vi "Navigation_Main_position_testing april 18th.vi"() -> ()   [LabVIEW 2015]
uses:
  <vilib>/myRIO/Instrument Drivers/Onboard IO/PWM/typedefs/PWM Reference.ctl
  <vilib>/myRIO/Common/Instrument Driver Framework/Utilities/typedefs/myRIO Generic Hardware Reference.ctl
  <vilib>/myRIO/Common/Instrument Driver Framework/Utilities/typedefs/Hardware Version Enum.ctl
  <vilib>/myRIO/Common/Instrument Driver Framework/Utilities/typedefs/myRIO v1.0 Reference.ctl
  <vilib>/myRIO/Common/Instrument Driver Framework/Utilities/typedefs/Generic FPGA Reference.ctl
  <vilib>/myRIO/Common/Instrument Driver Framework/myRIO v1.0/PWM/typedefs/PWM Channels Enum.ctl
  <vilib>/myRIO/Instrument Drivers/Onboard IO/PWM/typedefs/PWM Configuration.ctl
  <vilib>/userdefined/High Color/nirio_resource_hc.ctl
  <vilib>/myRIO/Common/Instrument Driver Framework/myRIO v1.0/PWM/vis/myRIO v1.1 Open PWM.vi
  <vilib>/myRIO/Common/Instrument Driver Framework/Utilities/vis/Validate Channels.vi
  <vilib>/myRIO/Common/Instrument Driver Framework/myRIO v1.0/PWM/vis/myRIO v1.0 Reserve PWM.vi
  <vilib>/myRIO/Common/Instrument Driver Framework/myRIO v1.0/PWM/vis/myRIO v1.0 Build MUX Configuration PWM.vi
  <vilib>/myRIO/Common/Instrument Driver Framework/myRIO v1.0/Resource Manager/vis/myRIO v1.0 Reserve Channel List.vi
  <vilib>/myRIO/Common/Instrument Driver Framework/myRIO v1.0/Resource Manager/vis/myRIO v1.0 Create Configuration List.vi
  <vilib>/myRIO/Common/Instrument Driver Framework/myRIO v1.0/Resource Manager/vis/myRIO v1.0 Reserve Channel.vi
  <vilib>/myRIO/Common/Instrument Driver Framework/myRIO v1.0/Resource Manager/vis/myRIO v1.0 Unreserve Channel.vi
  <vilib>/myRIO/Common/Instrument Driver Framework/myRIO v1.0/Resource Manager/vis/myRIO v1.0 Build Mutex Name.vi
  <vilib>/FPGAPlugInAG/myRIO-1900/niLvFpga_Open_myRIO-1900.vi
  <vilib>/rvi/interface/common/dynamic/niFpgaDynamicAddResources.vi
  <vilib>/myRIO/Common/Instrument Driver Framework/Utilities/vis/FPGA Ref Manager.vi
  <vilib>/Utility/error.llb/Error Cluster From Error Code.vi
  <vilib>/myRIO/Common/Instrument Driver Framework/Utilities/vis/Ref Counter.vi
  <vilib>/rvi/errors/niLvFpgaAdjustHostInterfaceError.vi
  <vilib>/Utility/VariantDataType/GetNumericInfo.vi
  <vilib>/myRIO/Common/Instrument Driver Framework/myRIO v1.0/myRIO v1.1 Open.vi
  <vilib>/myRIO/Common/Instrument Driver Framework/Utilities/vis/IO Manager.vi
  <vilib>/myRIO/Common/Instrument Driver Framework/Utilities/vis/Configuration Manager.vi
  <vilib>/myRIO/Common/Instrument Driver Framework/myRIO v1.0/Resource Manager/vis/myRIO v1.0 Configure IO.vi
  <vilib>/myRIO/Common/Instrument Driver Framework/myRIO v1.0/myRIO v1.0 Close.vi
  <vilib>/myRIO/Common/Instrument Driver Framework/myRIO v1.0/PWM/vis/myRIO v1.0 Write PWM.vi
  <vilib>/addons/control/pid/pid.llb/PID (DBL).vi
  <vilib>/rvi/interface/nirviOpenFPGA/nirviOpenFPGA.xnode
  Navi/E/FPGA Bitfiles/NavigationProjec_FPGATarget2_FPGAMainNavigati_PWPHW8gwDxI.lvbitx
  <vilib>/rvi/interface/nirviReadWriteControl/nirviReadWriteControl.xnode
  <vilib>/myRIO/Instrument Drivers/Onboard IO/PWM/vis/myRIO PWM Open.xnode
  <vilib>/myRIO/Instrument Drivers/Onboard IO/PWM/PWM.lvlib
  <vilib>/myRIO/Instrument Drivers/Utilities/Utilities.lvlib
  NiFpgaLv.dll
  <vilib>/rvi/interface/Simulation/niFpgaSimulationCallBeginRW.vi
  <vilib>/addons/control/pid/NI_PID_pid.lvlib
panel:
  out "right 2":dbl
  out "left 2":dbl
  in  "right ctrl":dbl min=-0.133 max=0.133 step=0.01
  in  "left ctrl":dbl min=-0.133 max=0.133 step=0.01
  in  "reset start position":bool=TRUE
  in  "theta goal":dbl=10.0
  in  "y goal":dbl=10.0
  out "stop switch":dbl=1.0
  out "distance to goal":dbl
  out "loc_y":dbl
  out "loc_x":dbl
  out "loc_theta":dbl
  out "start y":dbl
  out "start angle":dbl=1.0
  out "start x":dbl=1.0
  in  "set start position":bool=TRUE
  out "goal reached":bool=TRUE
  out "x/y":dbl
  out "scale":dbl=1.0
  in  "x goal":dbl=10.0
  in  "L Desired Input Velocity (ft/s) 4":dbl(knob) scale=-4.0..4.0
  in  "R Min Linear Velocity (ft/s)  2":dbl=-2.0 format="%#_13g"
  in  "L Min Linear Velocity (ft/s) 9":dbl=-2.0 format="%#_13g"
  in  "R Max Linear Velocity (ft/s) 5":dbl=2.0 format="%#_13g"
  in  "L Max Linear Velocity (ft/s) 5":dbl=2.0 format="%#_13g"
  in  "R Desired Input Velocity (ft/s) 5":dbl(knob) scale=-4.0..4.0
  out "left":dbl
  out "right":dbl
  out "left wheels actual pwm":dbl
  in  "stop 3":bool
  out "left pwm":dbl(graph)
  out "dt out (s) 3":dbl format="%.3f"
  in  "output range 3":cluster{"output high":dbl, "output low":dbl}={"output high"=0.13333, "output low"=-0.13333} {"output low" format="%.6f"; "output high" format="%.5f"}
  in  "PID gains 3":T1={"proportional gain (Kc)"=0.002, "integral time (Ti, min)"=7e-07, "derivative time (Td, min)"=0.0} {"derivative time (Td, min)" format="%.8f"; "integral time (Ti, min)" format="%.8f"; "proportional gain (Kc)" format="%.8f"}
  out "desired pwm 2":dbl
  out "feedback 2":dbl
  out ".not. x? 3":bool
  out "Elapsed Time (s) 2":dbl caption="Elapsed Time (s)"
  out "x traveled 2":dbl
  out "y traveled 2":dbl
  out "avg 124":dbl
  out "avg 457":dbl
  out "psi dot 2":dbl
  out "distance traveled 2":dbl
  out "y dot 2":dbl
  out "x dot 2":dbl
  out "x position 2":dbl
  out "y position 2":dbl
  out "reset x y 2":dbl
  out "Tick Count(mSec) 2":u32 caption="Tick Count(mSec)"
  in  "start y 2":dbl=3.0
  in  "start x 2":dbl=1.0
  out "right wheels actual pwm":dbl
  in  "stop 2":bool
  out "right pwm":dbl(graph)
  out "dt out (s) 2":dbl format="%.3f"
  in  "output range 2":cluster{"output high":dbl, "output low":dbl}={"output high"=0.13333, "output low"=-0.13333} {"output low" format="%.6f"; "output high" format="%.5f"}
  in  "PID gains 2":T1={"proportional gain (Kc)"=0.002, "integral time (Ti, min)"=7e-07, "derivative time (Td, min)"=0.0} {"derivative time (Td, min)" format="%.8f"; "integral time (Ti, min)" format="%.8f"; "proportional gain (Kc)" format="%.8f"}
  out "desired pwm":dbl
  out "feedback":dbl
  out ".not. x? 2":bool
  out "Elapsed Time (s)":dbl
  out "LF Rot Velocity (rot/s)":dbl
  out "LM Rot Velocity (rot/s)":dbl
  out "LR Rot Velocity (rot/s)":dbl
  out "RR Rot Velocity (rot/s)":dbl
  out "RM Linear Velocity (rot/s)":dbl
  out "RF Linear Velocity (rot/s)":dbl
  in  "Encoder Reset":bool
  out "SYS.SELECTA":u8 format="%08b"
  out "ENC.B_c.CNTR":i32
  out "ENC.B_b.CNTR":i32
  out "ENC.B_a.CNTR":i32
  out "ENC.A_c.CNTR":i32
  out "ENC.A_b.CNTR":i32
  out "ENC.A_a.CNTR":i32
  in  "R Min Linear Velocity (ft/s)":dbl=-2.0 format="%#_13g"
  in  "R Max Linear Velocity (ft/s)":dbl=2.0 format="%#_13g"
  in  "L Min Linear Velocity (ft/s)":dbl=-2.0 format="%#_13g"
  in  "L Max Linear Velocity (ft/s)":dbl=2.0 format="%#_13g"
  out "Current Rot Velocity (rot/s)":T2(graph)
  # "starts the loop"
  # "Motor Control Parameters"
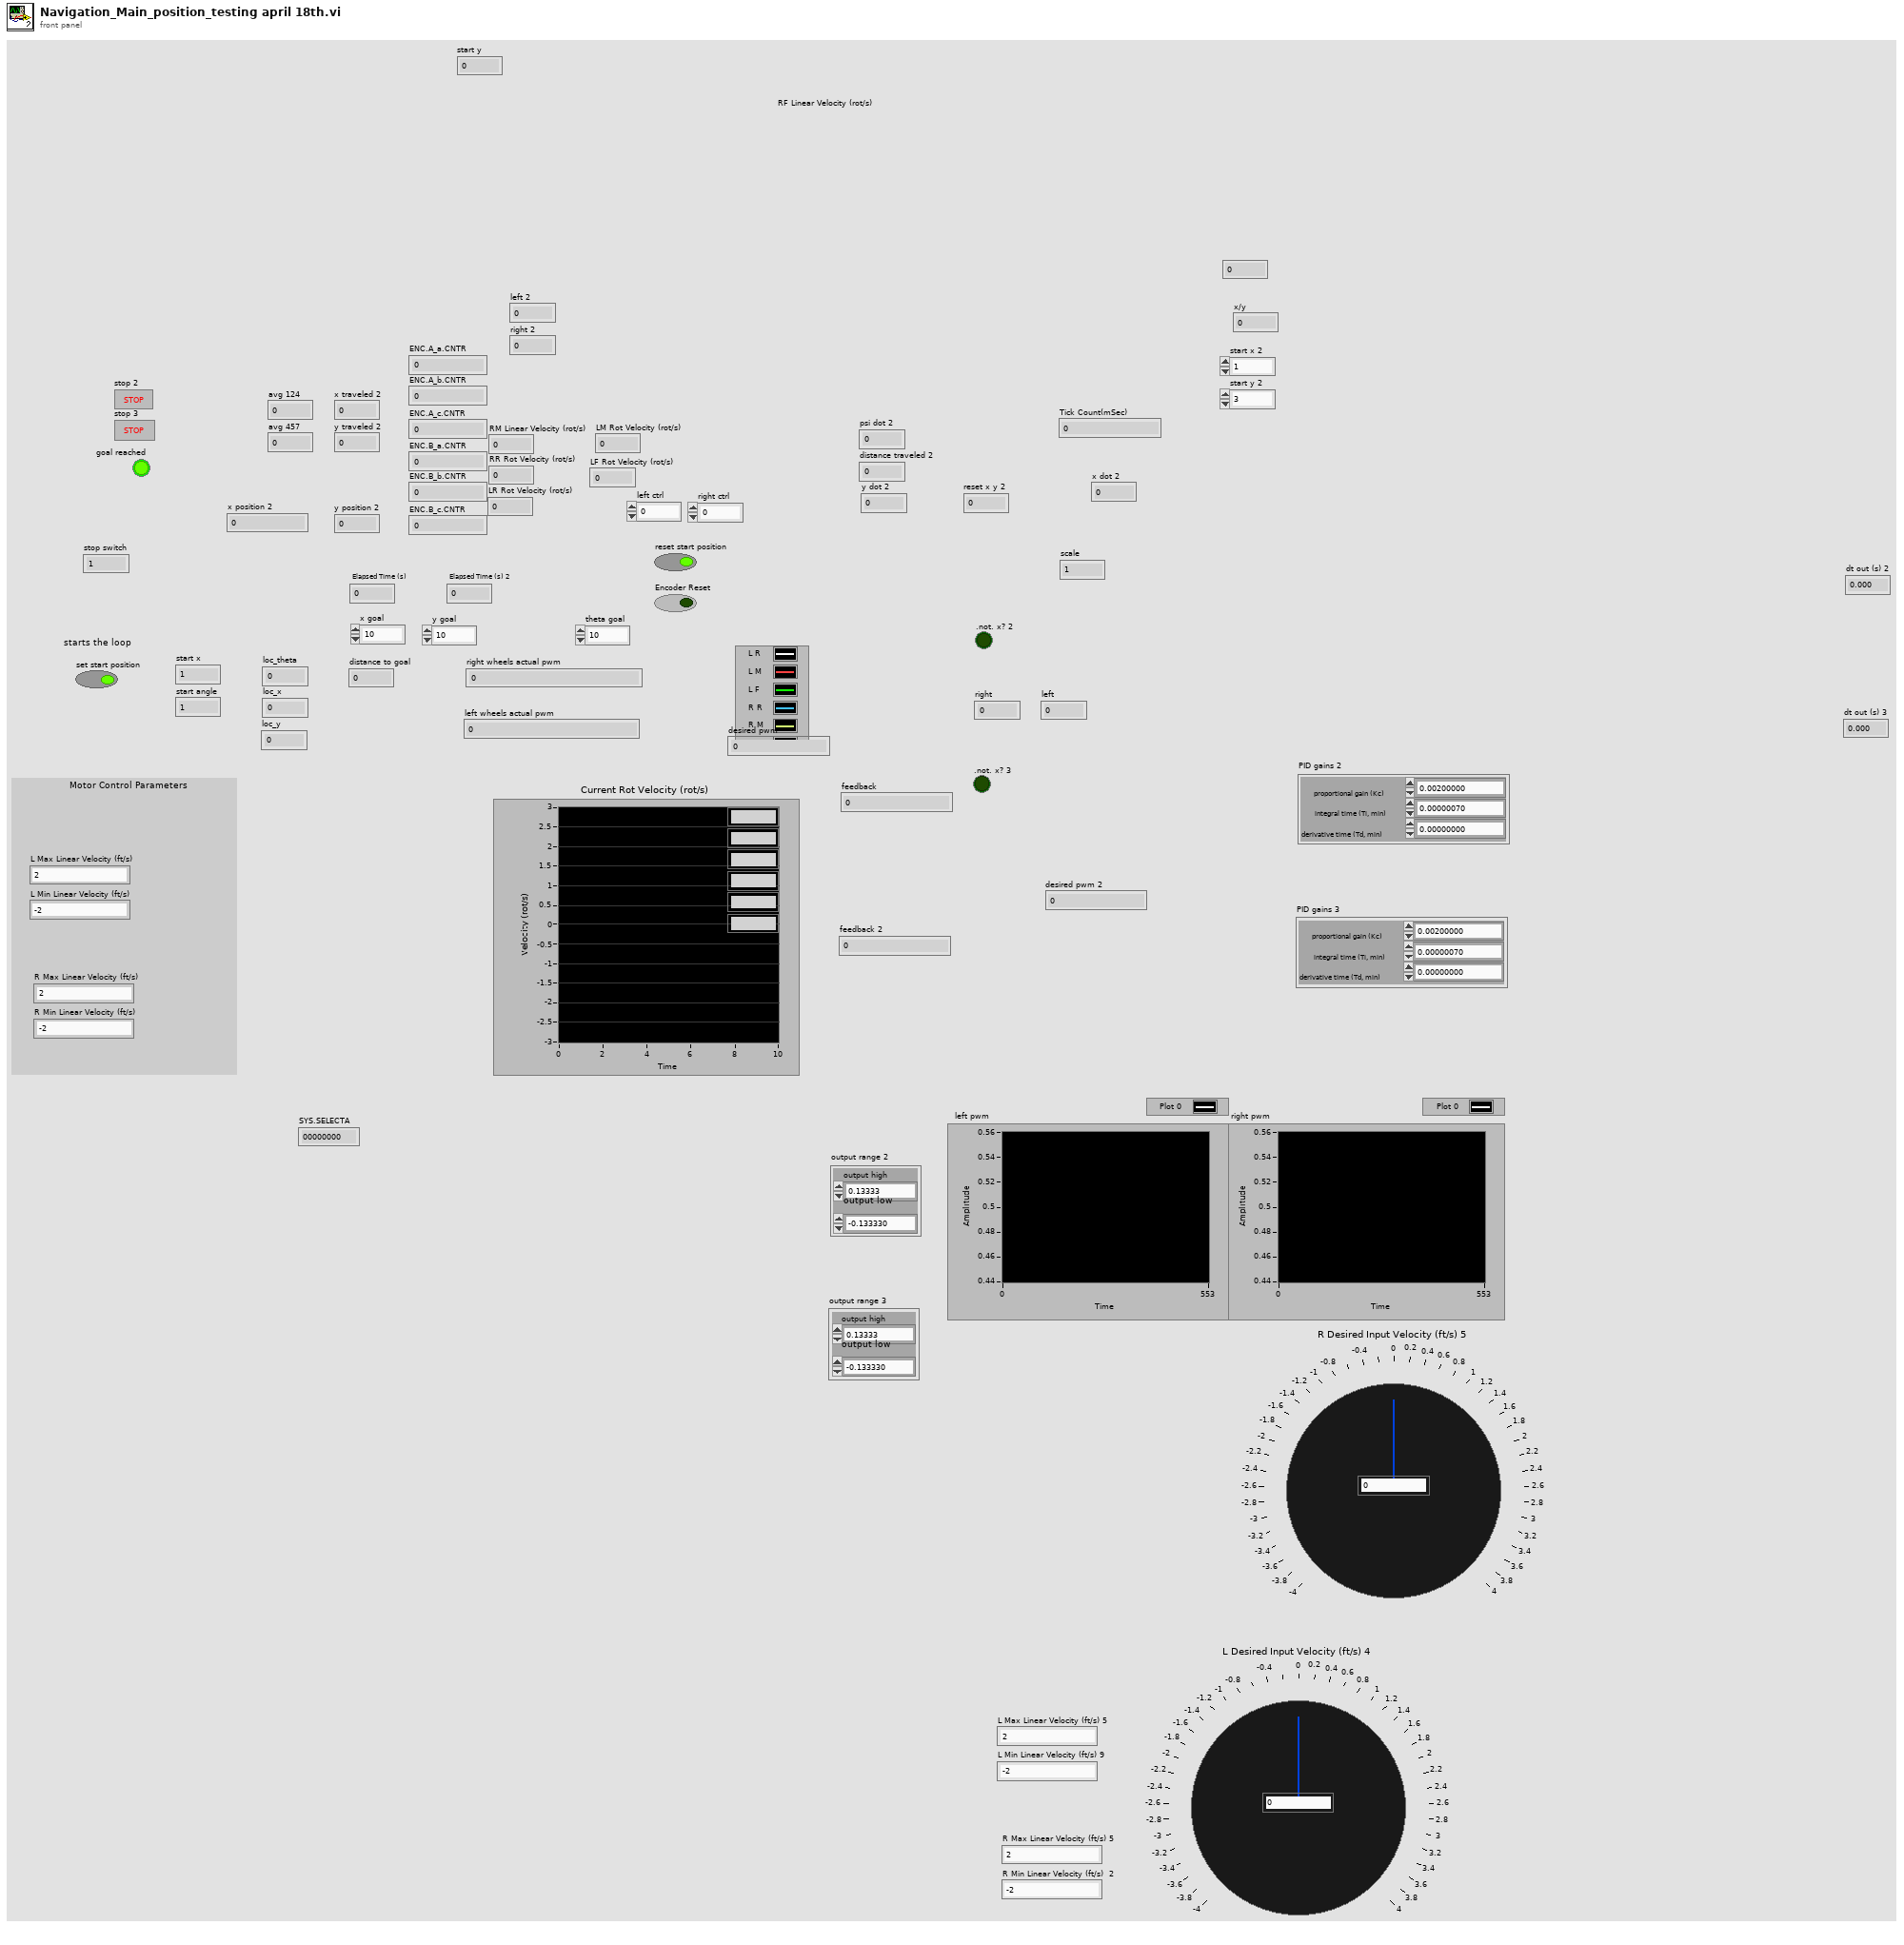
[diagram p1: front panel]
types:
  T1 = cluster{"proportional gain (Kc)":dbl, "integral time (Ti, min)":dbl, "derivative time (Td, min)":dbl}
  T2 = cluster{"Rotational Velocity (RPS)":dbl, "Rotational Velocity (RPS)":dbl, "Rotational Velocity (RPS)":dbl, "Rotational Velocity (RPS)":dbl, "Rotational Velocity (RPS)":dbl, "Rotational Velocity (RPS)":dbl}
  T3 = typedef "nirio_resource_hc.ctl" = tag
  T4 = typedef "Hardware Version Enum.ctl" = enum16{"Unknown", "myRIO-1900", "myRIO-1950", "roboRIO"}
  T5 = typedef "PWM.lvlib/PWM Reference.ctl" = cluster{"myRIO Reference":T6, "PWM Channels Enum":T9, "PWM Configuration":T10}
  T6 = typedef "myRIO Generic Hardware Reference.ctl" = cluster{"myRIO Model":T4, "myRIO Hardware Reference":T7}
  T7 = typedef "myRIO v1.0 Reference.ctl" = cluster{"Generic FPGA Reference":T8, "Allow multiple opens":bool}
  T8 = typedef "Generic FPGA Reference.ctl" = refnum<k20>
  T9 = typedef "PWM Channels Enum.ctl" = enum16{"Not Connected", "C/PWM0", "C/PWM1", "A/PWM0", "A/PWM1", "A/PWM2", "B/PWM0", "B/PWM1", "B/PWM2", "PWM/PWM0", "PWM/PWM1", "PWM/PWM2", "PWM/PWM3", "PWM/PWM4", "PWM/PWM5", "PWM/PWM6", "PWM/PWM7", "PWM/PWM8", "PWM/PWM9"}
  T10 = typedef "PWM.lvlib/PWM Configuration.ctl" = cluster{"Frequency":dbl, "Duty Cycle":dbl}
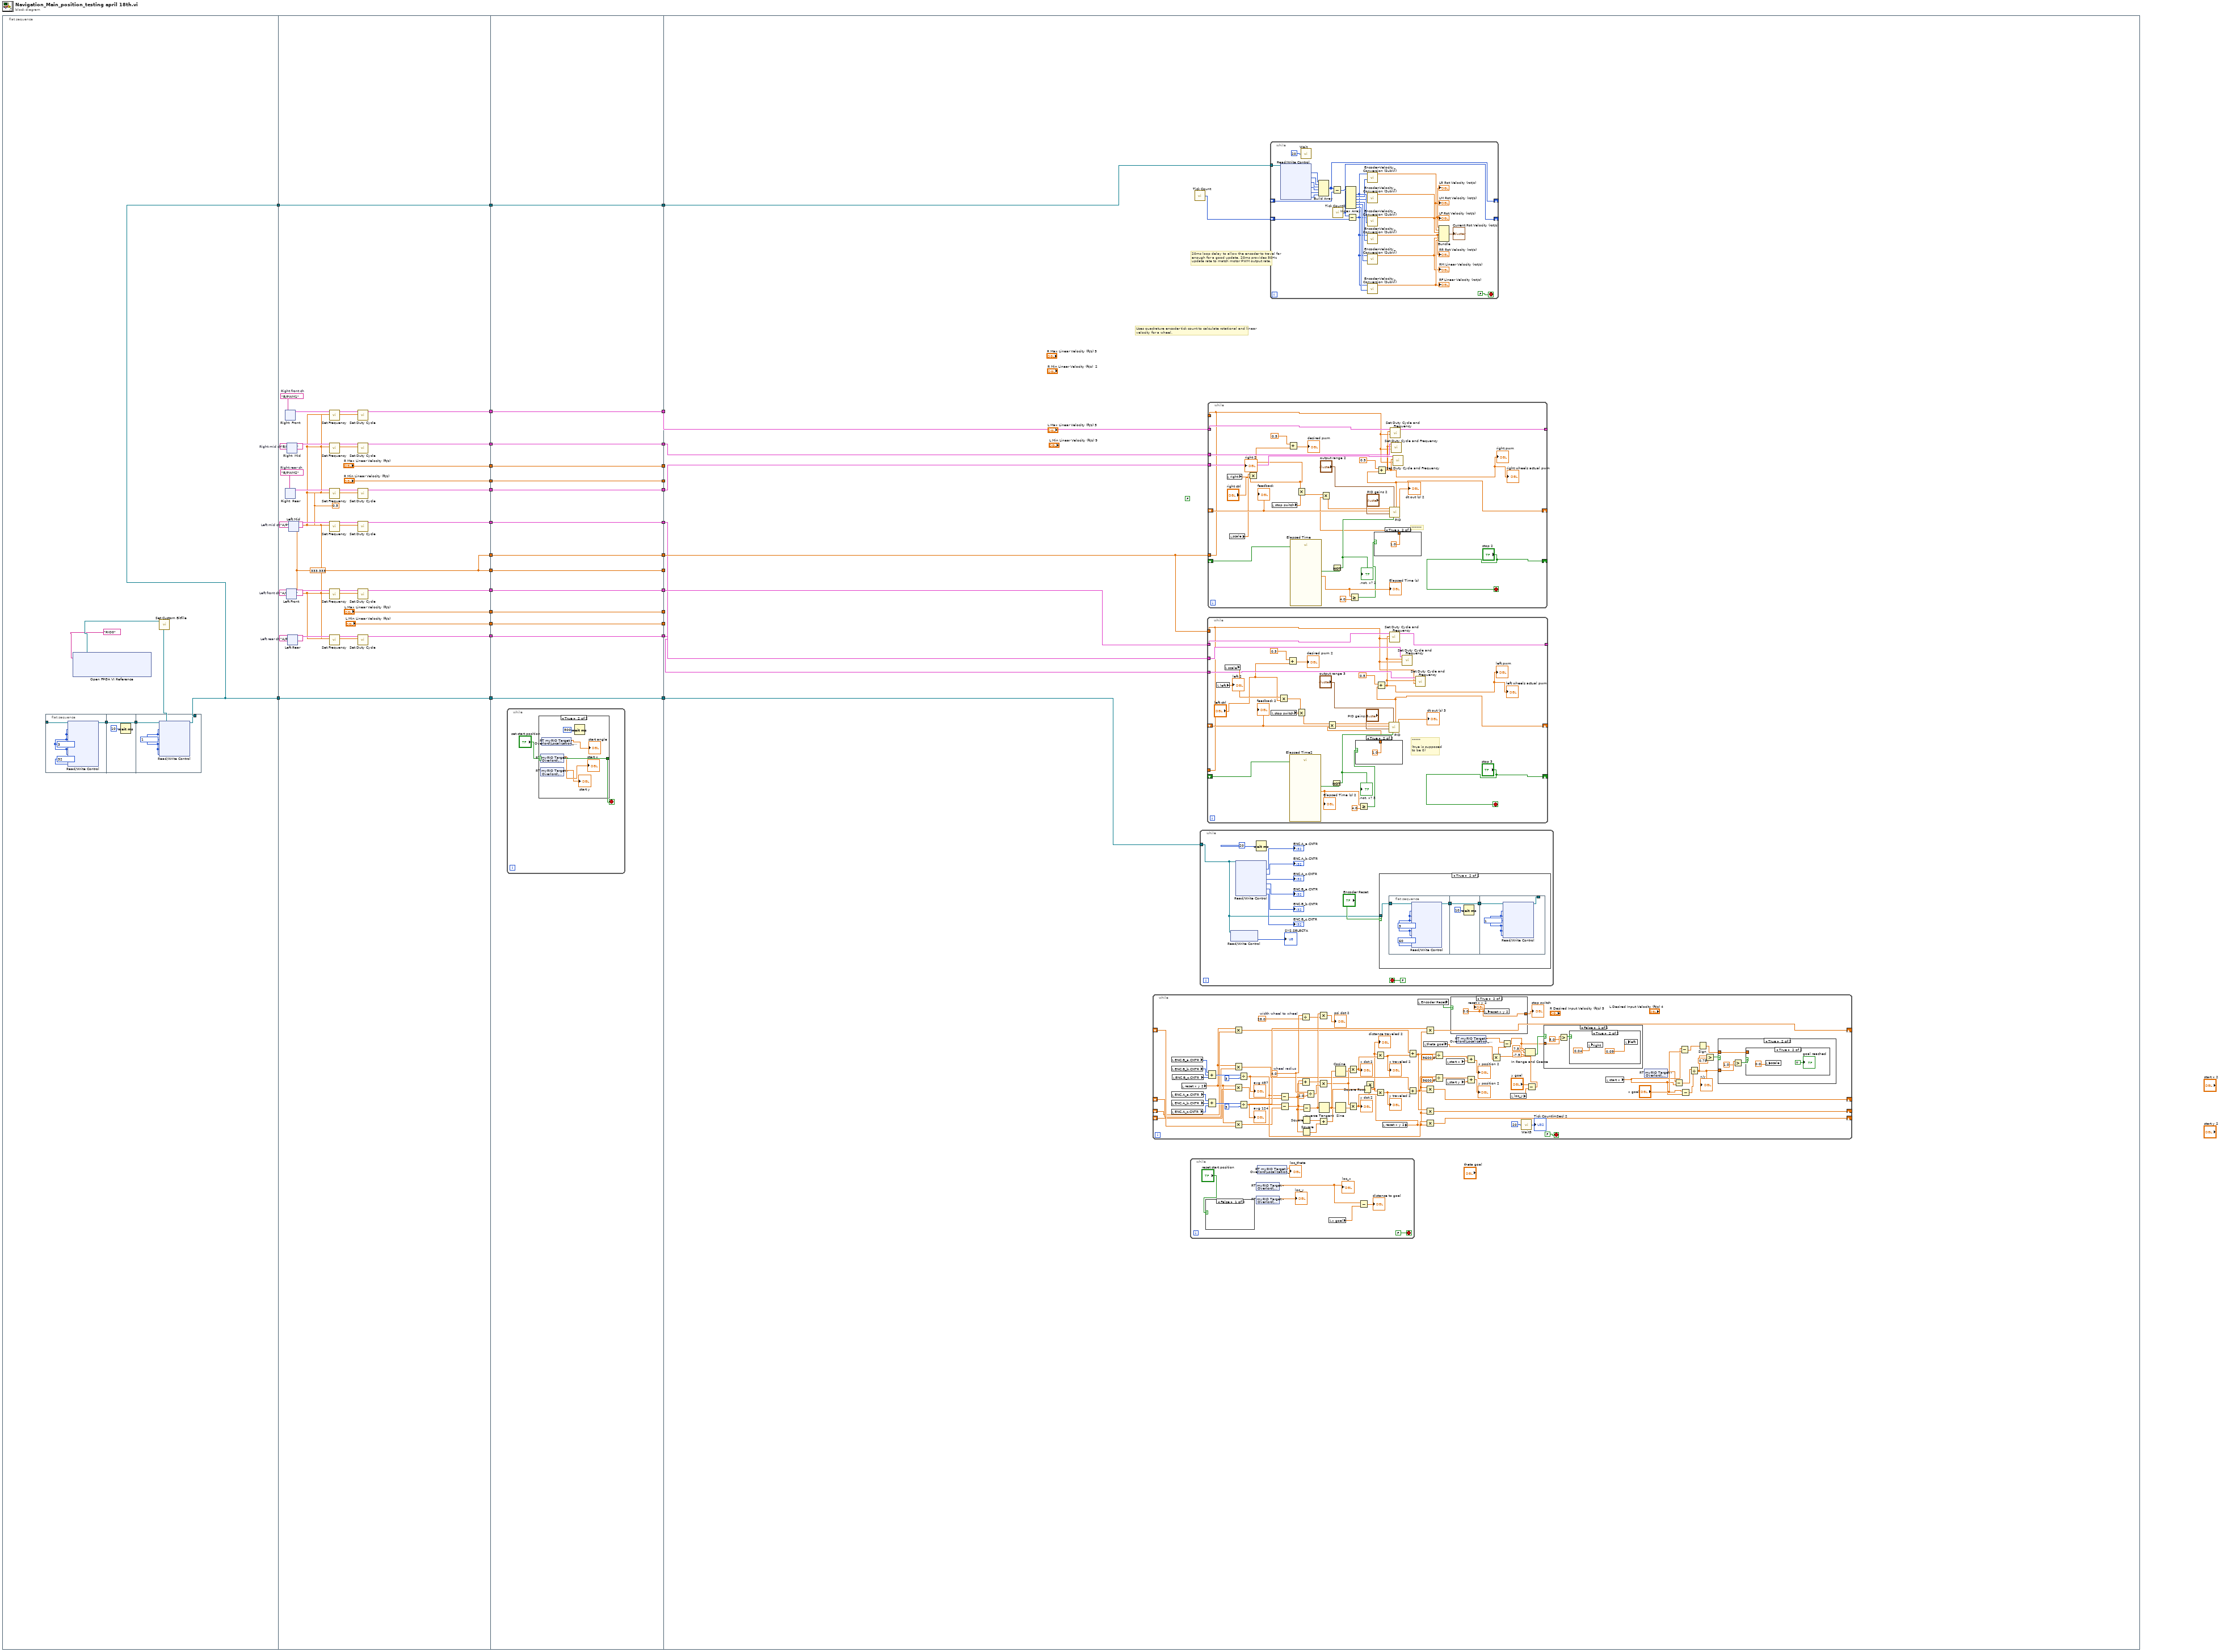
[diagram p0: block diagram]
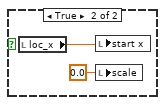
[diagram p3: hidden frame]
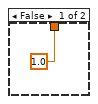
[diagram p4: hidden frame]
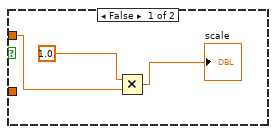
[diagram p5: hidden frame]
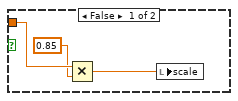
[diagram p6: hidden frame]
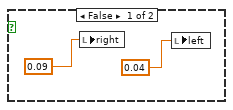
[diagram p7: hidden frame]
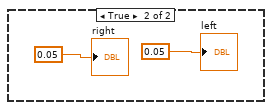
[diagram p8: hidden frame]
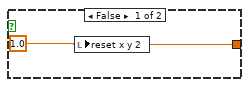
[diagram p9: hidden frame]
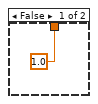
[diagram p10: hidden frame]
diagram:
  n1 = flat-sequence {
    tunnel: [w33] -> w30
    tunnel: [w33] -> w29
    tunnel: [w46] -> w28
    tunnel: [w61] -> w26
    tunnel: [w57] -> w24
    tunnel: [w56] -> w22
    tunnel: [w55] -> w20
    tunnel: [w54] -> w18
    tunnel: [w53] -> w16
    tunnel: ["L Max Linear Velocity (ft/s)"] -> w14
    tunnel: ["L Min Linear Velocity (ft/s)"] -> w12
    tunnel: ["R Max Linear Velocity (ft/s)"] -> w10
    tunnel: ["R Min Linear Velocity (ft/s)"] -> w8
    tunnel: [w48] -> w6
    tunnel: w30 -> [w47]
    tunnel: [w47] -> w4
    tunnel: w29 -> [w48]
    tunnel: [w46] -> w2
    tunnel: w28 -> [w187]
    tunnel: [w187] -> w27
    tunnel: w26 -> [w186]
    tunnel: [w186] -> w25
    tunnel: w24 -> [w185]
    tunnel: [w185] -> w23
    tunnel: w22 -> [w184]
    tunnel: [w184] -> w21
    tunnel: w20 -> [w183]
    tunnel: [w183] -> w19
    tunnel: w18 -> [w182]
    tunnel: [w182] -> w17
    tunnel: w16 -> [w181]
    tunnel: [w181] -> w15
    tunnel: w14 -> [w180]
    tunnel: [w180] -> w13
    tunnel: w12 -> [w179]
    tunnel: [w179] -> w11
    tunnel: w10 -> [w178]
    tunnel: [w178] -> w9
    tunnel: w8 -> [w177]
    tunnel: [w177] -> w7
    tunnel: w6 -> [w176]
    tunnel: [w176] -> w5
    tunnel: w4 -> [w175]
    tunnel: [w175] -> w3
    tunnel: w2 -> [w174]
    tunnel: [w174] -> w1
    tunnel: w27 -> [_]
    tunnel: w25 -> [w195]
    tunnel: w23 -> [w201]
    tunnel: w21 -> [w198]
    tunnel: w19 -> [w197]
    tunnel: w17 -> [w196]
    tunnel: w15 -> [w200]
    tunnel: w13 -> [_]
    tunnel: w11 -> [_]
    tunnel: w9 -> [_]
    tunnel: w7 -> [_]
    tunnel: w5 -> [w203]
    tunnel: w3 -> [w202]
    tunnel: w1 -> [w199]
    frame #0 {
      n2 = flat-sequence {
        tunnel: w34 -> [w39]
        tunnel: [w37] -> w36
        tunnel: w36 -> [w41]
        tunnel: [w41] -> w35
        tunnel: w35 -> [w44]
        tunnel: [w43] -> w33
        frame #0 {
          w38 = u8 32 ("SYS.SELECTA")
          w40 = u8 3 ("ENC.B_c.CNFG")
          n3 = xnode "Read/Write Control"("FPGA VI Reference In"=w39, "ENC.A_a.CNFG"=w40, "ENC.A_b.CNFG"=w40, "ENC.A_c.CNFG"=w40, "ENC.B_a.CNFG"=w40, "ENC.B_b.CNFG"=w40, "ENC.B_c.CNFG"=w40, "SYS.SELECTA"=w38, "SYS.SELECTB"=w38) -> ("FPGA VI Reference Out"=w37:refnum<k20>)  [unwired: 1 in, 1 out]
        }
        frame #1 {
          n4 = Wait (ms)(milliseconds to wait=u32 10) -> ()  [unwired: 1 out]
        }
        frame #2 {
          w45 = u8 1 ("ENC.B_c.CNFG")
          n5 = xnode "Read/Write Control"("FPGA VI Reference In"=w44, "ENC.A_a.CNFG"=w45, "ENC.A_b.CNFG"=w45, "ENC.A_c.CNFG"=w45, "ENC.B_a.CNFG"=w45, "ENC.B_b.CNFG"=w45, "ENC.B_c.CNFG"=w45) -> ("FPGA VI Reference Out"=w43:refnum<k20>)  [unwired: 1 in, 1 out]
        }
      }
      n6 = xnode "Open FPGA VI Reference"("resource name"=tag "RIO0") -> ("FPGA VI Reference Out"=w32:refnum<k20>)  [unwired: 1 in, 1 out]
      n7 = call <vilib>:"Set Custom Bitfile.vi"("Custom FPGA Reference In"=w32) -> ("Custom FPGA Reference Out"=w34:refnum<k20>)  [unwired: 9 in, 1 out]
    }
    frame #1 {
      w58 = 0.5 ("Duty Cycle")
      w46 = 333.333 ("Frequency [Hz]")
      w72 = tag "B/PWM2"  # Right rear ch
      w73 = tag "B/PWM0"  # Right mid ch
      w74 = tag "B/PWM1"  # Right front ch
      w75 = tag "A/PWM2"  # Left rear ch
      w76 = tag "A/PWM1"  # Left mid ch
      w77 = tag "A/PWM0"  # Left front ch
      n8 = xnode "Right  Front"("Channel Name"=w74) -> ("PWM Ref Out"=w68:T5)  [unwired: 2 in, 1 out]
      n9 = xnode "Right  Rear"("Channel Name"=w72) -> ("PWM Ref Out"=w66:T5)  [unwired: 2 in, 1 out]
      n10 = xnode "Left Front"("Channel Name"=w77) -> ("PWM Ref Out"=w71:T5)  [unwired: 2 in, 1 out]
      n11 = xnode "Right  Mid"("Channel Name"=w73) -> ("PWM Ref Out"=w67:T5)  [unwired: 2 in, 1 out]
      n12 = xnode "Left Rear"("Channel Name"=w75) -> ("PWM Ref Out"=w69:T5)  [unwired: 2 in, 1 out]
      n13 = xnode "Left Mid"("Channel Name"=w76) -> ("PWM Ref Out"=w70:T5)  [unwired: 2 in, 1 out]
      n14 = call <vilib>:"Set Frequency.vi"("Frequency [Hz]"=w46, "PWM Ref In"=w68) -> ("PWM Ref Out"=w62:T5)  [unwired: 7 in, 1 out]
      n15 = call <vilib>:"Set Frequency.vi"("Frequency [Hz]"=w46, "PWM Ref In"=w67) -> ("PWM Ref Out"=w63:T5)  [unwired: 7 in, 1 out]
      n16 = call <vilib>:"Set Frequency.vi"("Frequency [Hz]"=w46, "PWM Ref In"=w66) -> ("PWM Ref Out"=w64:T5)  [unwired: 7 in, 1 out]
      n17 = call <vilib>:"Set Frequency.vi"("Frequency [Hz]"=w46, "PWM Ref In"=w70) -> ("PWM Ref Out"=w59:T5)  [unwired: 7 in, 1 out]
      n18 = call <vilib>:"Set Frequency.vi"("Frequency [Hz]"=w46, "PWM Ref In"=w71) -> ("PWM Ref Out"=w65:T5)  [unwired: 7 in, 1 out]
      n19 = call <vilib>:"Set Frequency.vi"("Frequency [Hz]"=w46, "PWM Ref In"=w69) -> ("PWM Ref Out"=w60:T5)  [unwired: 7 in, 1 out]
      n20 = call <vilib>:"Set Duty Cycle.vi"("Duty Cycle"=w58, "PWM Ref In"=w62) -> ("PWM Ref Out"=w57:T5)  [unwired: 7 in, 1 out]
      n21 = call <vilib>:"Set Duty Cycle.vi"("Duty Cycle"=w58, "PWM Ref In"=w63) -> ("PWM Ref Out"=w56:T5)  [unwired: 7 in, 1 out]
      n22 = call <vilib>:"Set Duty Cycle.vi"("Duty Cycle"=w58, "PWM Ref In"=w64) -> ("PWM Ref Out"=w55:T5)  [unwired: 7 in, 1 out]
      n23 = call <vilib>:"Set Duty Cycle.vi"("Duty Cycle"=w58, "PWM Ref In"=w59) -> ("PWM Ref Out"=w54:T5)  [unwired: 7 in, 1 out]
      n24 = call <vilib>:"Set Duty Cycle.vi"("Duty Cycle"=w58, "PWM Ref In"=w65) -> ("PWM Ref Out"=w53:T5)  [unwired: 7 in, 1 out]
      n25 = call <vilib>:"Set Duty Cycle.vi"("Duty Cycle"=w58, "PWM Ref In"=w60) -> ("PWM Ref Out"=w61:T5)  [unwired: 7 in, 1 out]
    }
    frame #2 {
      n26 = while {
        stop <- w188 stop-if-true
        n27 = case shown="True" "set start position" {
          selector: "set start position" -> [_ w194]
          tunnel: [_ w194] -> w188
          frame False {
          }
          frame True {
            n28 = shared-variable "RT myRIO Target - Overlord\\Localization_Variables_r0.lvlib\\loc_x"() -> (→"start x":dbl)  [unwired: 1 in, 1 out]
            n29 = shared-variable "RT myRIO Target - Overlord\\Localization_Variables_r0.lvlib\\loc_y"() -> (→"start y":dbl)  [unwired: 1 in, 1 out]
            n30 = shared-variable "RT myRIO Target - Overlord\\Localization_Variables_r0.lvlib\\loc_theta"() -> (→"start angle":dbl)  [unwired: 1 in, 1 out]
            n31 = Wait (ms)(milliseconds to wait=u32 500) -> ()  [unwired: 1 out]
          }
        }
      }
    }
    frame #3 {
      (unwired) FALSE
      # "Uses quadrature encoder tick count to calculate rotational and linear velocity for a wheel."
      # "20ms loop delay to allow the encoder to travel far enough for a good update. 20ms provides 50Hz update rate to match motor PWM output rate."
      n32 = while {
        shift-right: [w277] -> _
        shift-left: _ -> [w315]
        shift-right: [w274] -> _
        shift-left: _ -> [w314]
        shift-right: [w276] -> _
        shift-left: _ -> [w289]
        shift-right: [w275] -> _
        shift-left: _ -> [w288]
        stop <- FALSE stop-if-true
        w310 = 28.0  # width wheel to wheel
        w311 = 4.0  # wheel radius
        n33 = local read "ENC.B_a.CNTR"() -> (w320:i32)
        n34 = local read "ENC.B_b.CNTR"() -> (w319:i32)
        n35 = local read "ENC.A_a.CNTR"() -> (w323:i32)
        n36 = local read "ENC.A_b.CNTR"() -> (w322:i32)
        n37 = local read "ENC.A_c.CNTR"() -> (w321:i32)
        n38 = local read "ENC.B_c.CNTR"() -> (w318:i32)
        n39 = local read "reset x y 2"() -> (w273:dbl)
        n40 = Compound Arithmetic op=ADD(w320, w319, w318) -> (w326:i32)
        n41 = Compound Arithmetic op=ADD(w323, w322, w321) -> (w327:i32)
        n42 = Multiply(x=w273, y=w288) -> (x*y=w279:dbl)
        n43 = Multiply(x=w273, y=w289) -> (x*y=w280:dbl)
        n44 = Multiply(x=w273, y=w314) -> (x*y=w278:dbl)
        n45 = Multiply(x=w273, y=w315) -> (x*y=w281:dbl)
        n46 = Divide(x=w326, y=3) -> (x/y=w313:dbl)
        "avg 457" <- w313
        n47 = Divide(x=w327, y=3) -> (x/y=w316:dbl)
        "avg 124" <- w316
        n48 = Subtract(x=w313, y=w278) -> (x-y=w303:dbl)
        n49 = Subtract(x=w316, y=w281) -> (x-y=w304:dbl)
        n50 = Divide(x=w311, y=w310) -> (x/y=w306:dbl)
        n51 = Add(x=w304, y=w303) -> (x+y=w308:dbl)
        n52 = Square(x=w304) -> (x^2=w301:dbl)
        n53 = Square(x=w303) -> (x^2=w302:dbl)
        n54 = Subtract(x=w304, y=w303) -> (x-y=w307:dbl)
        n55 = Divide(x=w311, y=2.0) -> (x/y=w309:dbl)
        n56 = Multiply(x=w307, y=w306) -> (x*y=→"psi dot 2":dbl)
        n57 = Multiply(x=w308, y=w309) -> (x*y=w297:dbl)
        n58 = Add(x=w301, y=w302) -> (x+y=w300:dbl)
        n59 = Inverse Tangent(1:w307) -> (0:w305:dbl)
        n60 = Cosine(x=w305) -> (cos(x)=w298:dbl)
        n61 = Sine(x=w305) -> (sin(x)=w299:dbl)
        n62 = Multiply(x=w297, y=w298) -> (x*y=w295:dbl)
        "x dot 2" <- w295
        n63 = Multiply(x=w297, y=w299) -> (x*y=w296:dbl)
        "y dot 2" <- w296
        n64 = Square Root(x=w300) -> (sqrt(x)=w294:dbl)
        n65 = local read "reset x y 2"() -> (w271:dbl)
        n66 = Multiply(x=w294, y=w271) -> (x*y=w272:dbl)
        "distance traveled 2" <- w272
        n67 = Multiply(x=w272, y=w295) -> (x*y=w293:dbl)
        "x traveled 2" <- w293
        n68 = Multiply(x=w272, y=w296) -> (x*y=w292:dbl)
        "y traveled 2" <- w292
        n69 = Add(x=w279, y=w293) -> (x+y=w291:dbl)
        n70 = Add(x=w280, y=w292) -> (x+y=w283:dbl)
        n71 = local read "Encoder Reset"() -> (w270:bool)
        n72 = local read "theta goal"() -> (w251:dbl)
        n73 = Multiply(x=w316, y=w271) -> (x*y=w277:dbl)
        n74 = Multiply(x=w271, y=w283) -> (x*y=w276:dbl)
        n75 = Multiply(x=w291, y=w271) -> (x*y=w275:dbl)
        n76 = Multiply(x=w313, y=w271) -> (x*y=w274:dbl)
        n77 = Divide(x=w291, y=9600.0) -> (x/y=w286:dbl)
        n78 = Divide(x=w283, y=9600.0) -> (x/y=w287:dbl)
        n79 = local read "start x"() -> (w284:dbl)
        n80 = local read "start y"() -> (w285:dbl)
        n81 = case shown="True" w270 {
          tunnel: [w350 w351] -> w252
          frame False {
            w350 = 1.0
            n82 = local write "reset x y 2"(w350) -> ()
          }
          frame True {
            w351 = 0.0
            n83 = local write "reset x y 2"(w351) -> ()
            "reset x y 2" <- w351
          }
        }
        "stop switch" <- w252
        n84 = shared-variable "RT myRIO Target - Overlord\\Localization_Variables_r0.lvlib\\loc_theta"() -> (w250:dbl)  [unwired: 1 in, 1 out]
        n85 = Add(x=w286, y=w284) -> (x+y=→"x position 2":dbl)
        n86 = Add(x=w287, y=w285) -> (x+y=→"y position 2":dbl)
        n87 = local read "loc_y"() -> (w246:dbl)
        n88 = call "Wait3"("Count(mSec)"=u32 20) -> ("Tick Count(mSec)"=→"Tick Count(mSec) 2":u32)
        n89 = Subtract(x="y goal", y=w246) -> (x-y=w245:dbl)
        n90 = Multiply(x=w245, y=w251) -> (x*y=w248:dbl)
        n91 = Subtract(x=w250, y=w248) -> (x-y=w249:dbl)
        n92 = In Range and Coerce(upper limit=7.5, x=w249, lower limit=-7.5) -> (In Range?=w264:bool)  [unwired: 1 out]
        n93 = case shown="False" w264 {
          tunnel: w249 -> [w343 _]
          frame False {
            n94 = Greater?(x=w343, y=5.0) -> (0:w341:bool)
            n95 = case shown="True" w341 {
              frame False {
                n96 = local write "right"(0.09) -> ()
                n97 = local write "left"(0.04) -> ()
              }
              frame True {
                n98 = local write "right"(0.04) -> ()
                n99 = local write "left"(0.09) -> ()
              }
            }
          }
          frame True {
            "right" <- 0.05
            "left" <- 0.05
          }
        }
        n100 = local read "start x"() -> (w255:dbl)
        n101 = shared-variable "RT myRIO Target - Overlord\\Localization_Variables_r0.lvlib\\loc_x"() -> (w253:dbl)  [unwired: 1 in, 1 out]
        n102 = Subtract(x=w253, y=w255) -> (x-y=w260:dbl)
        n103 = Subtract(x=w255, y="x goal") -> (x-y=w257:dbl)
        n104 = Subtract(x="x goal", y=w255) -> (x-y=w259:dbl)
        n105 = Divide(x=w260, y=w259) -> (x/y=w261:dbl)
        "x/y" <- w261
        n106 = Sign(1:w257) -> (0:w256:dbl)
        n107 = Greater?(x=w261, y=0.75) -> (0:w262:bool)
        n108 = case shown="True" w262 {
          tunnel: w261 -> [_ w335]
          tunnel: w256 -> [w330 w332]
          frame False {
            n109 = Multiply(x=1.0, y=w330) -> (x*y=→"scale":dbl)
          }
          frame True {
            n110 = Greater?(x=w335, y=1.0) -> (0:w333:bool)
            n111 = case shown="True" w333 {
              tunnel: w332 -> [w338 _]
              frame False {
                n112 = Multiply(x=w338, y=0.85) -> (x*y=w336:dbl)
                n113 = local write "scale"(w336) -> ()
              }
              frame True {
                n114 = local write "scale"(0.0) -> ()
                "goal reached" <- TRUE
              }
            }
          }
        }
      }
      n115 = while {
        stop <- FALSE stop-if-true
        n116 = case shown="False" "reset start position" {
          frame False {
          }
          frame True {
            n117 = local read "loc_x"() -> (w213:dbl)
            n118 = local write "start x"(w213) -> ()
            n119 = local write "scale"(0.0 ("scale")) -> ()
          }
        }
        n120 = shared-variable "RT myRIO Target - Overlord\\Localization_Variables_r0.lvlib\\loc_x"() -> (w209:dbl)  [unwired: 1 in, 1 out]
        "loc_x" <- w209
        n121 = shared-variable "RT myRIO Target - Overlord\\Localization_Variables_r0.lvlib\\loc_y"() -> (→"loc_y":dbl)  [unwired: 1 in, 1 out]
        n122 = shared-variable "RT myRIO Target - Overlord\\Localization_Variables_r0.lvlib\\loc_theta"() -> (→"loc_theta":dbl)  [unwired: 1 in, 1 out]
        n123 = local read "x goal"() -> (w208:dbl)
        n124 = Subtract(x=w209, y=w208) -> (x-y=→"distance to goal":dbl)
      }
      n125 = call "Tick Count"() -> ("Tick Count(uSec)"=w204:u32)
      n126 = while {
        tunnel: w203 -> [w383]
        stop <- FALSE stop-if-true
        n127 = xnode "Read/Write Control"("FPGA VI Reference In"=w383) -> ("SYS.SELECTA"=→"SYS.SELECTA":u8)  [unwired: 1 in, 2 out]
        n128 = xnode "Read/Write Control"("FPGA VI Reference In"=w383) -> ("ENC.A_a.CNTR"=→"ENC.A_a.CNTR":u32, "ENC.A_b.CNTR"=→"ENC.A_b.CNTR":u32, "ENC.A_c.CNTR"=→"ENC.A_c.CNTR":u32, "ENC.B_a.CNTR"=→"ENC.B_a.CNTR":u32, "ENC.B_b.CNTR"=→"ENC.B_b.CNTR":u32, "ENC.B_c.CNTR"=→"ENC.B_c.CNTR":u32)  [unwired: 1 in, 2 out]
        n129 = Wait (ms)(milliseconds to wait=u32 20) -> ()  [unwired: 1 out]
        n130 = case shown="True" "Encoder Reset" {
          tunnel: w383 -> [_ w394]
          frame False {
          }
          frame True {
            n131 = flat-sequence {
              tunnel: w394 -> [w399]
              tunnel: [w397] -> w396
              tunnel: w396 -> [w401]
              tunnel: [w401] -> w395
              tunnel: w395 -> [w404]
              tunnel: [w403] -> _
              frame #0 {
                w398 = u8 60 ("SYS.SELECTA")
                w400 = u8 3 ("ENC.B_c.CNFG")
                n132 = xnode "Read/Write Control"("FPGA VI Reference In"=w399, "ENC.A_a.CNFG"=w400, "ENC.A_b.CNFG"=w400, "ENC.A_c.CNFG"=w400, "ENC.B_a.CNFG"=w400, "ENC.B_b.CNFG"=w400, "ENC.B_c.CNFG"=w400, "SYS.SELECTA"=w398, "SYS.SELECTB"=w398) -> ("FPGA VI Reference Out"=w397:refnum<k20>)  [unwired: 1 in, 1 out]
              }
              frame #1 {
                n133 = Wait (ms)(milliseconds to wait=u32 10) -> ()  [unwired: 1 out]
              }
              frame #2 {
                w405 = u8 1 ("ENC.B_c.CNFG")
                n134 = xnode "Read/Write Control"("FPGA VI Reference In"=w404, "ENC.A_a.CNFG"=w405, "ENC.A_b.CNFG"=w405, "ENC.A_c.CNFG"=w405, "ENC.B_a.CNFG"=w405, "ENC.B_b.CNFG"=w405, "ENC.B_c.CNFG"=w405) -> ("FPGA VI Reference Out"=w403:refnum<k20>)  [unwired: 1 in, 1 out]
              }
            }
          }
        }
      }
      n135 = while {
        tunnel: w200 -> [w241]
        tunnel: [w242] -> _
        tunnel: w199 -> [w227]
        shift-right: [w226] -> _
        shift-left: _ -> [w237]
        shift-right: ["stop 3"] -> _
        shift-left: _ -> [w219]
        tunnel: [w227] -> _
        tunnel: w196 -> [w230]
        tunnel: w195 -> [w229]
        stop <- "stop 3" stop-if-true
        # "*****\n\n(true is supposed\nto be 0)"
        n136 = local read "left"() -> (→"left 2":dbl)
        n137 = local read "scale"() -> (w231:dbl)
        n138 = local read "stop switch"() -> (w223:dbl)
        n139 = Multiply(x=w231, y="left ctrl") -> (x*y=w225:dbl)
        n140 = Add(x=0.5, y="left ctrl") -> (x+y=→"desired pwm 2":dbl)
        n141 = call "Elapsed Time2"("Reset"=w219) -> ("Elapsed Time (s)"=w218:dbl, "Time has Elapsed"=w222:bool)  [unwired: 11 in, 6 out]
        "Elapsed Time (s) 2" <- w218
        n142 = Multiply(x=w225, y=w223) -> (x*y=w224:dbl)
        n143 = Not(x=w222) -> (.not. x?=w235:bool)
        ".not. x? 3" <- w235
        n144 = Greater Or Equal?(x=w218, y=4.0) -> (x >= y?=w216:bool)
        n145 = case shown="True" w216 {
          tunnel: [1.0 1.0] -> w220
          frame False {
          }
          frame True {
          }
        }
        n146 = Multiply(x=w224, y=w220) -> (x*y=w221:dbl)
        n147 = call-poly <vilib>:"PID.vi"("reinitialize? (F)"=w235, "output range"="output range 3", "PID gains"="PID gains 3", "process variable"=w237, "setpoint"=w221) -> ("dt out (s)"=→"dt out (s) 3":dbl, "output"=w226:dbl)  [unwired: 5 in]
        n148 = Add(x=0.5, y=w226) -> (x+y=w228:dbl)
        "left wheels actual pwm" <- w228
        "left pwm" <- w228
        n149 = call <vilib>:"Set Duty Cycle and Frequency.vi"("Frequency [Hz]"=w227, "Duty Cycle"=w228, "PWM Ref In"=w241) -> ("PWM Ref Out"=w242:T5)  [unwired: 6 in, 1 out]
        n150 = call <vilib>:"Set Duty Cycle and Frequency.vi"("Frequency [Hz]"=w227, "Duty Cycle"=w228, "PWM Ref In"=w230) -> ()  [unwired: 6 in, 2 out]
        n151 = call <vilib>:"Set Duty Cycle and Frequency.vi"("Frequency [Hz]"=w227, "Duty Cycle"=w228, "PWM Ref In"=w229) -> ()  [unwired: 6 in, 2 out]
        "feedback 2" <- w237
      }
      n152 = while {
        tunnel: w201 -> [w379]
        tunnel: [w380] -> _
        tunnel: [w365] -> _
        shift-right: [w364] -> _
        shift-left: _ -> [w375]
        shift-right: ["stop 2"] -> _
        shift-left: _ -> [w358]
        tunnel: w199 -> [w365]
        tunnel: w198 -> [w368]
        tunnel: w197 -> [w367]
        stop <- "stop 2" stop-if-true
        # "******"
        n153 = local read "right"() -> (→"right 2":dbl)
        n154 = local read "scale"() -> (w369:dbl)
        n155 = Multiply(x=w369, y="right ctrl") -> (x*y=w363:dbl)
        n156 = local read "stop switch"() -> (w361:dbl)
        n157 = Add(x=0.5, y=w363) -> (x+y=→"desired pwm":dbl)
        n158 = call "Elapsed Time"("Reset"=w358) -> ("Elapsed Time (s)"=w357:dbl, "Time has Elapsed"=w355:bool)  [unwired: 11 in, 6 out]
        "Elapsed Time (s)" <- w357
        n159 = Multiply(x=w363, y=w361) -> (x*y=w362:dbl)
        n160 = Not(x=w355) -> (.not. x?=w373:bool)
        ".not. x? 2" <- w373
        n161 = Greater Or Equal?(x=w357, y=4.0) -> (x >= y?=w354:bool)
        n162 = case shown="True" w354 {
          tunnel: [1.0 1.0] -> w359
          frame False {
          }
          frame True {
          }
        }
        n163 = Multiply(x=w362, y=w359) -> (x*y=w360:dbl)
        n164 = call-poly <vilib>:"PID.vi"("reinitialize? (F)"=w373, "output range"="output range 2", "PID gains"="PID gains 2", "process variable"=w375, "setpoint"=w360) -> ("dt out (s)"=→"dt out (s) 2":dbl, "output"=w364:dbl)  [unwired: 5 in]
        n165 = Add(x=0.5, y=w364) -> (x+y=w366:dbl)
        "right wheels actual pwm" <- w366
        "right pwm" <- w366
        n166 = call <vilib>:"Set Duty Cycle and Frequency.vi"("Frequency [Hz]"=w365, "Duty Cycle"=w366, "PWM Ref In"=w379) -> ("PWM Ref Out"=w380:T5)  [unwired: 6 in, 1 out]
        n167 = call <vilib>:"Set Duty Cycle and Frequency.vi"("Frequency [Hz]"=w365, "Duty Cycle"=w366, "PWM Ref In"=w368) -> ()  [unwired: 6 in, 2 out]
        n168 = call <vilib>:"Set Duty Cycle and Frequency.vi"("Frequency [Hz]"=w365, "Duty Cycle"=w366, "PWM Ref In"=w367) -> ()  [unwired: 6 in, 2 out]
        "feedback" <- w375
      }
      n169 = while {
        shift-right: [w424] -> _
        shift-left: _ -> [w423]
        shift-right: [w421] -> _
        shift-left: w204 -> [w420]
        tunnel: w202 -> [w431]
        stop <- FALSE stop-if-true
        n170 = xnode "Read/Write Control"("FPGA VI Reference In"=w431) -> ("ENC.A_a.CNTR"=w430:u32, "ENC.A_b.CNTR"=w429:u32, "ENC.A_c.CNTR"=w428:u32, "ENC.B_a.CNTR"=w427:u32, "ENC.B_b.CNTR"=w426:u32, "ENC.B_c.CNTR"=w425:u32)  [unwired: 1 in, 2 out]
        n171 = call "Wait"("Count(mSec)"=u32 20) -> ()  [unwired: 1 out]
        n172 = Build Array(w430, w429, w428, w427, w426, w425) -> (w424:u32[])
        n173 = Subtract(x=w424, y=w423) -> (x-y=w422:u32[])
        n174 = call "Tick Count2"() -> ("Tick Count(uSec)"=w421:u32)
        n175 = Index Array(array=w422) -> (element #1=w419:u32, element #2=w418:u32, element #3=w417:u32, element #4=w416:u32, element #5=w415:u32, element #6=w414:u32)  [unwired: 6 in]
        n176 = Subtract(x=w421, y=w420) -> (x-y=w413:u32)
        n177 = call "Encoder-Velocity_Conversion (SubVI).vi"("delta  Encoder Count"=w418, "dt (uSec)"=w413) -> ("Rotational Velocity (RPS)"=w408:dbl)  [unwired: 7 in, 2 out]
        "LM Rot Velocity (rot/s)" <- w408
        n178 = call "Encoder-Velocity_Conversion (SubVI).vi"("delta  Encoder Count"=w417, "dt (uSec)"=w413) -> ("Rotational Velocity (RPS)"=w407:dbl)  [unwired: 7 in, 2 out]
        "LF Rot Velocity (rot/s)" <- w407
        n179 = call "Encoder-Velocity_Conversion (SubVI).vi"("delta  Encoder Count"=w419, "dt (uSec)"=w413) -> ("Rotational Velocity (RPS)"=w409:dbl)  [unwired: 7 in, 2 out]
        "LR Rot Velocity (rot/s)" <- w409
        n180 = call "Encoder-Velocity_Conversion (SubVI).vi"("delta  Encoder Count"=w416, "dt (uSec)"=w413) -> ("Rotational Velocity (RPS)"=w406:dbl)  [unwired: 7 in, 2 out]
        "RR Rot Velocity (rot/s)" <- w406
        n181 = call "Encoder-Velocity_Conversion (SubVI).vi"("delta  Encoder Count"=w415, "dt (uSec)"=w413) -> ("Rotational Velocity (RPS)"=w410:dbl)  [unwired: 7 in, 2 out]
        "RM Linear Velocity (rot/s)" <- w410
        n182 = call "Encoder-Velocity_Conversion (SubVI).vi"("delta  Encoder Count"=w414, "dt (uSec)"=w413) -> ("Rotational Velocity (RPS)"=w411:dbl)  [unwired: 7 in, 2 out]
        "RF Linear Velocity (rot/s)" <- w411
        n183 = Bundle("Rotational Velocity (RPS)"=w409, "Rotational Velocity (RPS)"=w408, "Rotational Velocity (RPS)"=w407, "Rotational Velocity (RPS)"=w406, "Rotational Velocity (RPS)"=w410, "Rotational Velocity (RPS)"=w411) -> (→"Current Rot Velocity (rot/s)":T2)  [unwired: 1 in]
      }
    }
  }
